vi "Leader.vi"   [LabVIEW 2016]
uses:
  <vilib>/NXT/Block Support/NXT_TimerIndex.ctl
  <vilib>/NXT/Block Support/NXT_OutputPort.ctl
  <vilib>/NXT/Subs/MotorOutput.ctl
  <vilib>/NXT/Dual Mode Library/Sensors/Reset_Timer.vi
  <vilib>/NXT/Dual Mode Library/Sensors/Read_Timer.vi
  <vilib>/NXT/Dual Mode Library/Motors/ResetMotor.vi
  <vilib>/NXT/Dual Mode Library/Motors/Rotation.vi
  <vilib>/NXT/NXTIO Xnodes/NXTIONodeSubVIs/NXTMoveMotors.vi
  <vilib>/NXT/Dual Mode Library/Display/drawNumber_float.vi
  <vilib>/NXT/NXTIO Xnodes/NXTIONodeSubVIs/NXTStopMotors.vi
  <vilib>/NXT/Dual Mode Library/Display/drawText.vi
  <vilib>/NXT/Dual Mode Library/Display/drawNumber.vi
  <vilib>/NXT/Dual Mode Library/Display/drawText_Right.vi
  <vilib>/NXT/Subs/LVHSConnector.ctl
  <vilib>/NXT/NXTIO Xnodes/AddressXNode/NXTIOAddress.xnode
  <vilib>/NXT/NXTIO Xnodes/NXTIOXNode/NXTIO.xnode
  <vilib>/NXT/LegoClasses/BrickReference/BrickReference.lvclass
types:
  T1 = typedef "NXT_TimerIndex.ctl" = u8
  T2 = typedef "LVHSConnector.ctl" = refnum<class "BrickReference.lvclass">
  T3 = typedef "NXT_OutputPort.ctl" = u8
  T4 = typedef "MotorOutput.ctl" = u8
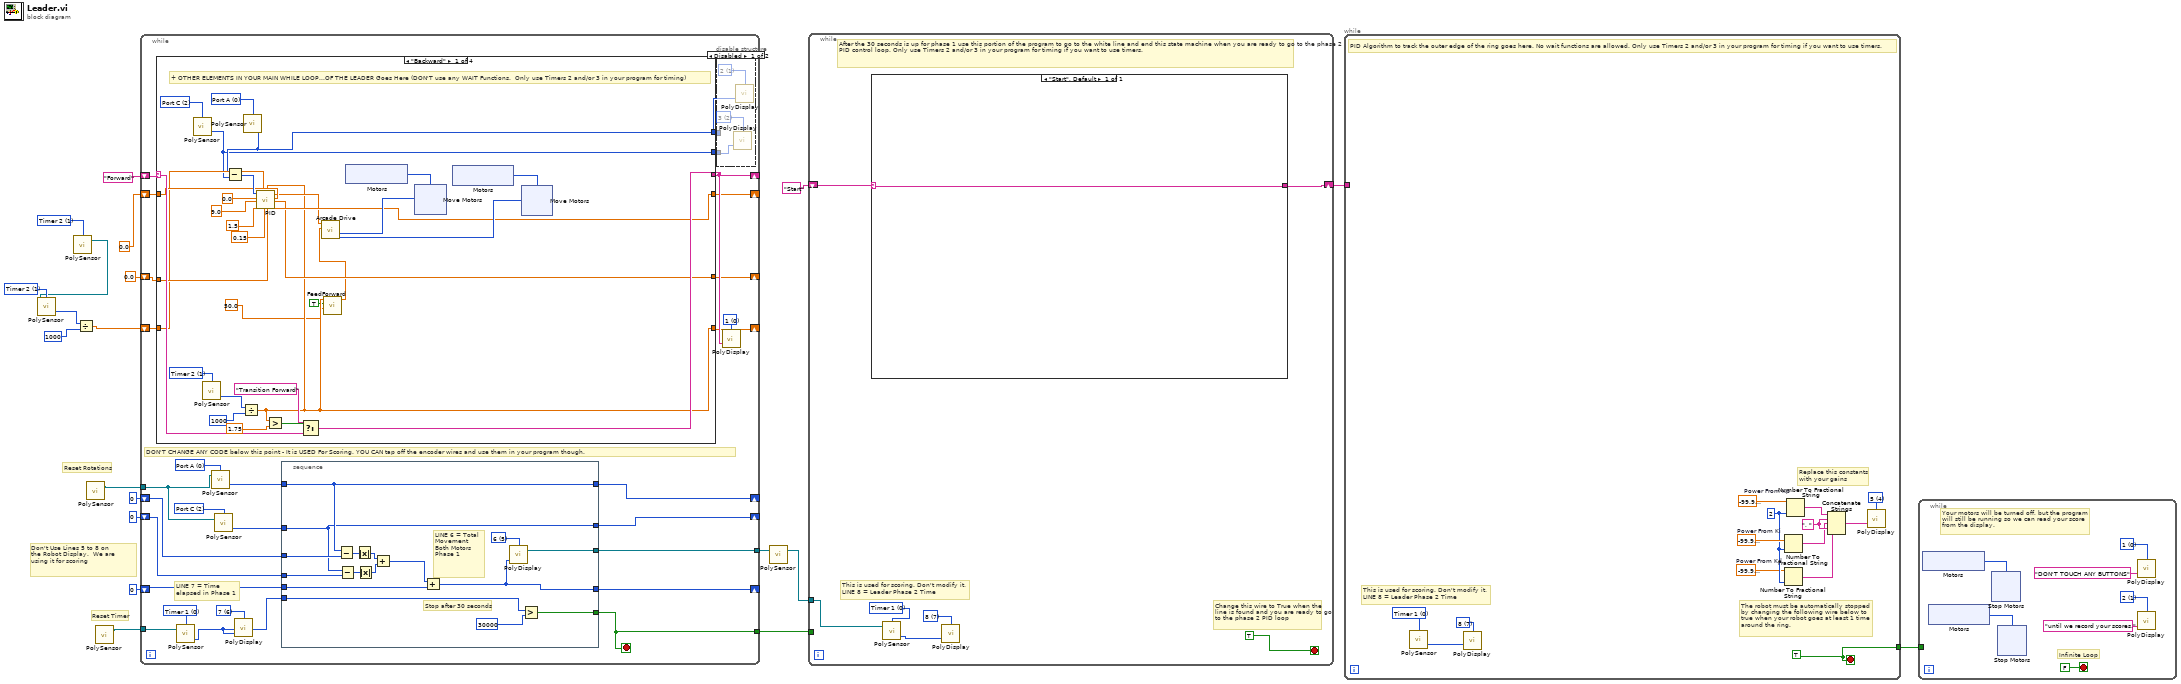
[diagram p0: block diagram]
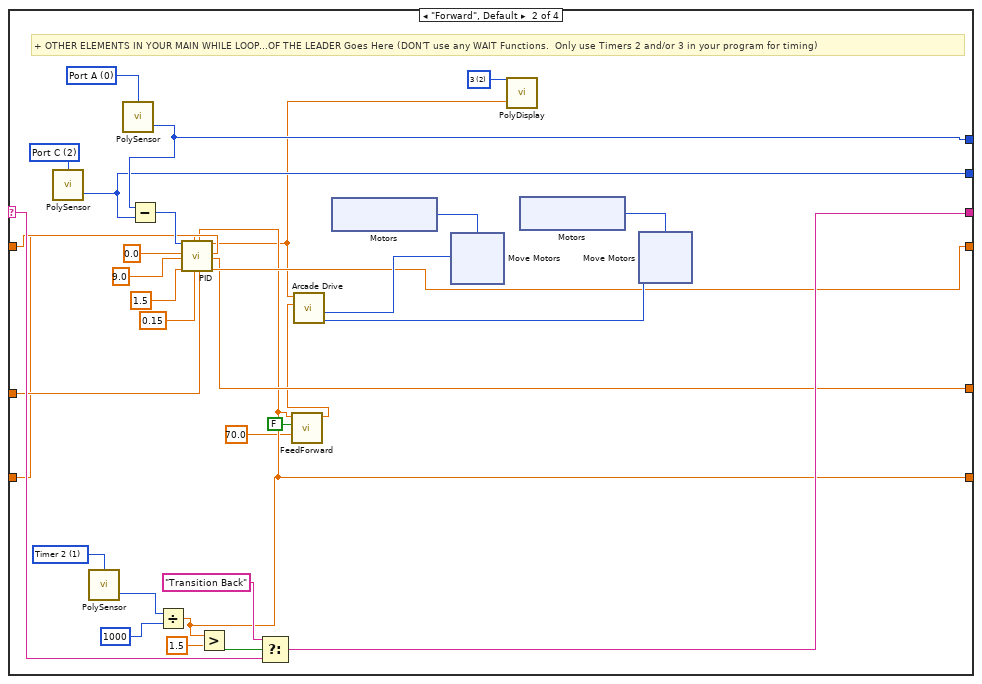
[diagram p3: hidden frame]
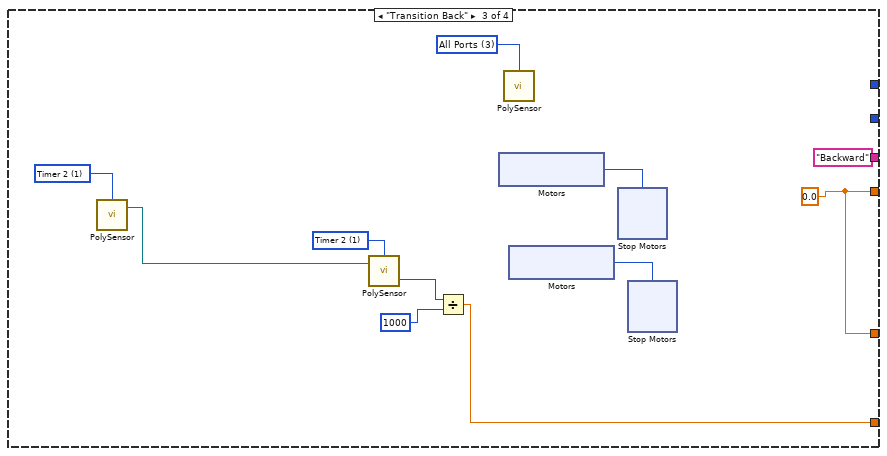
[diagram p4: hidden frame]
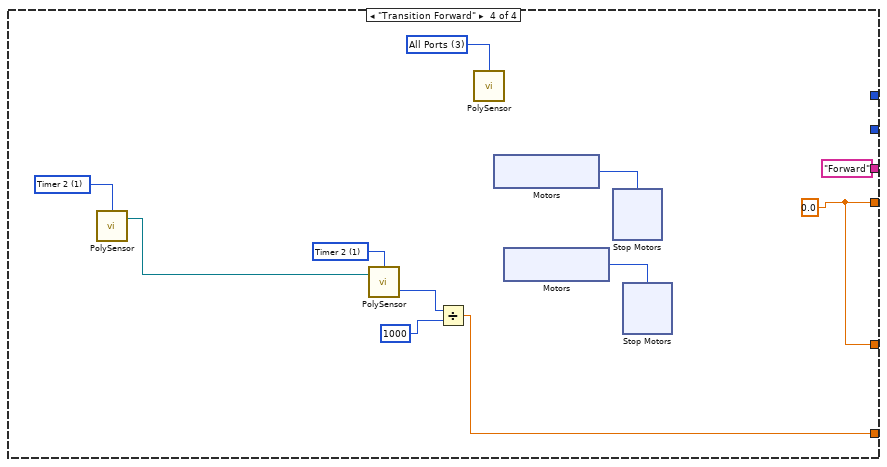
[diagram p5: hidden frame]
diagram:
  w4 = T1 1 items=["Timer 1", "Timer 2", "Timer 3"] ("Timer (Timer 1)")
  w8 = T1 1 items=["Timer 1", "Timer 2", "Timer 3"] ("Timer (Timer 1)")
  # "Don't Use Lines 5 to 8 on\nthe Robot Display.  We are \nusing it for scoring"
  # "Reset Timer"
  # "Reset Rotations"
  n1 = call-poly <vilib>:"PolySensor.vi"("Timer (Timer 1)"=w8) -> ("NXT/EV3"=w2:T2)  [unwired: 3 in]
  n2 = call-poly <vilib>:"PolySensor.vi"("NXT/EV3"=w2, "Timer (Timer 1)"=w4) -> ("Value (msec)"=w5:u32)  [unwired: 1 in, 1 out]
  n3 = Divide(x=w5, y=u32 1000) -> (x/y=w1:dbl)
  n4 = call-poly <vilib>:"PolySensor.vi"() -> ("NXT/EV3"=w16:T2)  [unwired: 4 in]
  n5 = call-poly <vilib>:"PolySensor.vi"() -> ("NXT/EV3"=w15:T2)  [unwired: 4 in]
  n6 = while {
    tunnel: w16 -> [w48]
    shift-right: [w40] -> _
    shift-left: 0 ("Angle of Rotation") -> [w42]
    shift-right: [w39] -> _
    shift-left: 0 ("Angle of Rotation") -> [w41]
    shift-right: [w46] -> _
    shift-left: 0 -> [w47]
    tunnel: w15 -> [w36]
    tunnel: [w45] -> w13
    shift-right: [w29] -> _
    shift-left: "Forward" -> [w38]
    tunnel: [w31] -> w12
    shift-right: [w27] -> _
    shift-left: 0.0 ("Accumulate In") -> [w28]
    shift-right: [w25] -> _
    shift-left: 0.0 ("Accumulate In") -> [w26]
    shift-right: [w23] -> _
    shift-left: w1 -> [w24]
    stop <- w45 stop-if-true
    w30 = i16 0 items=["1", "2", "3", "4", "5", "6", "7", "8", "9", "10", "11", "12"] ("Line")
    w33 = i16 6 items=["1", "2", "3", "4", "5", "6", "7", "8", "9", "10", "11", "12"] ("Line")
    w34 = T3 0 items=["Port A", "Port B", "Port C", "Port D"] ("Port (Port A)")
    w35 = T3 2 items=["Port A", "Port B", "Port C", "Port D"] ("Port (Port A)")
    w37 = T1 0 items=["Timer 1", "Timer 2", "Timer 3"] ("Timer (Timer 1)")
    # "DON'T CHANGE ANY CODE below this point - It is USED For Scoring. YOU CAN tap off the encoder wires and use them in your program though."
    # "LINE 7 = Time elapsed in Phase 1"
    n7 = case shown="\"Backward\"" w38 {
      selector: w38 -> [w78 w126 _ _]
      tunnel: [w79 w127 "Backward" ("t") "Forward" ("t")] -> w29
      tunnel: w28 -> [w65 w113 _ _]
      tunnel: [w63 w111 w156 w179] -> w27
      tunnel: w26 -> [w62 w110 _ _]
      tunnel: [w64 w112 w156 w179] -> w25
      tunnel: w24 -> [w61 w109 _ _]
      tunnel: [w57 w106 w151 w174] -> w23
      tunnel: [w60 w108 _ _] -> w22
      tunnel: [w59 w107 _ _] -> w21
      frame "Backward" {
        w73 = T3 2 items=["Port A", "Port B", "Port C", "Port D"] ("Port (Port A)")
        w74 = T3 0 items=["Port A", "Port B", "Port C", "Port D"] ("Port (Port A)")
        w81 = T1 1 items=["Timer 1", "Timer 2", "Timer 3"] ("Timer (Timer 1)")
        # "+ OTHER ELEMENTS IN YOUR MAIN WHILE LOOP...OF THE LEADER Goes Here (DON'T use any WAIT Functions.  Only use Timers 2 and/or 3 in your program for timing)"
        n8 = call-poly <vilib>:"PolySensor.vi"("Port (Port A)"=w73) -> ("Angle of Rotation"=w59:i32)  [unwired: 2 in, 1 out]
        n9 = call-poly <vilib>:"PolySensor.vi"("Timer (Timer 1)"=w81) -> ("Value (msec)"=w72:u32)  [unwired: 2 in, 1 out]
        n10 = Divide(x=w72, y=u32 1000) -> (x/y=w57:dbl)
        n11 = call-poly <vilib>:"PolySensor.vi"("Port (Port A)"=w74) -> ("Angle of Rotation"=w60:i32)  [unwired: 2 in, 1 out]
        n12 = Subtract(x=w60, y=w59) -> (x-y=w70:i32)
        n13 = call "PID.vi"("Sensor Input"=w70, "Setpoint"=0.0, "Kp"=9.0, "Ki"=1.5, "Prev Time"=w61, "Kd"=0.15, "Curr Time"=w57, "Accumulate In"=w65, "Previous Error"=w62) -> ("Output Val"=w58:dbl, "Accumulate Out"=w63:dbl, "Current Error"=w64:dbl)  [unwired: 5 in, 3 out]
        n14 = Greater?(x=w57, y=1.75) -> (0:w80:bool)
        n15 = Select(t="Transition Forward", s=w80, f=w78) -> (s? t:f=w79:string)
        n16 = call "FeedForward.vi"("FF Strength"=50.0, "backward?"=TRUE, "Current Time"=w57) -> ("f(t)"=w55:sgl)  [unwired: 8 in]
        n17 = call "Arcade Drive.vi"("Drive"=w55, "Rotate"=w58) -> ("Left Motor"=w75:i8, "Right Motor"=w76:i8)  [unwired: 8 in]
        n18 = xnode "Motors"() -> ("Motor"=w82:T3)
        n19 = xnode "Move Motors"("Power/Speed 1"=w76, "Motors"=w82) -> ()  [unwired: 1 in, 1 out]
        n20 = xnode "Motors"() -> ("Motor"=w83:T3)
        n21 = xnode "Move Motors"("Power/Speed 1"=w75, "Motors"=w83) -> ()  [unwired: 1 in, 1 out]
      }
      frame "Forward", Default {
        w103 = i16 2 items=["1", "2", "3", "4", "5", "6", "7", "8", "9", "10", "11", "12"] ("Line")
        w121 = T3 2 items=["Port A", "Port B", "Port C", "Port D"] ("Port (Port A)")
        w122 = T3 0 items=["Port A", "Port B", "Port C", "Port D"] ("Port (Port A)")
        w129 = T1 1 items=["Timer 1", "Timer 2", "Timer 3"] ("Timer (Timer 1)")
        # "+ OTHER ELEMENTS IN YOUR MAIN WHILE LOOP...OF THE LEADER Goes Here (DON'T use any WAIT Functions.  Only use Timers 2 and/or 3 in your program for timing)"
        n22 = call-poly <vilib>:"PolySensor.vi"("Port (Port A)"=w121) -> ("Angle of Rotation"=w107:i32)  [unwired: 2 in, 1 out]
        n23 = call-poly <vilib>:"PolySensor.vi"("Timer (Timer 1)"=w129) -> ("Value (msec)"=w120:u32)  [unwired: 2 in, 1 out]
        n24 = call-poly <vilib>:"PolySensor.vi"("Port (Port A)"=w122) -> ("Angle of Rotation"=w108:i32)  [unwired: 2 in, 1 out]
        n25 = Subtract(x=w108, y=w107) -> (x-y=w118:i32)
        n26 = Divide(x=w120, y=u32 1000) -> (x/y=w106:dbl)
        n27 = call "PID.vi"("Sensor Input"=w118, "Setpoint"=0.0, "Kp"=9.0, "Ki"=1.5, "Prev Time"=w109, "Kd"=0.15, "Curr Time"=w106, "Accumulate In"=w113, "Previous Error"=w110) -> ("Output Val"=w104:dbl, "Accumulate Out"=w111:dbl, "Current Error"=w112:dbl)  [unwired: 5 in, 3 out]
        n28 = Greater?(x=w106, y=1.5) -> (0:w128:bool)
        n29 = Select(t="Transition Back", s=w128, f=w126) -> (s? t:f=w127:string)
        n30 = call "FeedForward.vi"("FF Strength"=70.0, "backward?"=FALSE, "Current Time"=w106) -> ("f(t)"=w102:sgl)  [unwired: 8 in]
        n31 = call "Arcade Drive.vi"("Drive"=w102, "Rotate"=w104) -> ("Left Motor"=w123:i8, "Right Motor"=w124:i8)  [unwired: 8 in]
        n32 = xnode "Motors"() -> ("Motor"=w130:T3)
        n33 = xnode "Move Motors"("Power/Speed 1"=w124, "Motors"=w130) -> ()  [unwired: 1 in, 1 out]
        n34 = call-poly <vilib>:"PolyDisplay.vi"("number"=w104, "Line"=w103) -> ()  [unwired: 2 in, 1 out]
        n35 = xnode "Motors"() -> ("Motor"=w131:T3)
        n36 = xnode "Move Motors"("Power/Speed 1"=w123, "Motors"=w131) -> ()  [unwired: 1 in, 1 out]
      }
      frame "Transition Back" {
        w150 = T4 3 items=["Port A"=0, "Port B"=1, "Port C"=2, "Ports A & B"=4, "Ports A & C"=5, "Ports B & C"=6, "All Ports"=3] ("Port (All Ports)")
        w154 = T1 1 items=["Timer 1", "Timer 2", "Timer 3"] ("Timer (Timer 1)")
        w156 = 0.0 ("Accumulate In")
        w158 = T1 1 items=["Timer 1", "Timer 2", "Timer 3"] ("Timer (Timer 1)")
        n37 = call-poly <vilib>:"PolySensor.vi"("Timer (Timer 1)"=w158) -> ("NXT/EV3"=w152:T2)  [unwired: 3 in]
        n38 = call-poly <vilib>:"PolySensor.vi"("NXT/EV3"=w152, "Timer (Timer 1)"=w154) -> ("Value (msec)"=w153:u32)  [unwired: 1 in, 1 out]
        n39 = Divide(x=w153, y=u32 1000) -> (x/y=w151:dbl)
        n40 = xnode "Motors"() -> ("Motor"=w149:T3)
        n41 = call-poly <vilib>:"PolySensor.vi"("Port (All Ports)"=w150) -> ()  [unwired: 3 in, 1 out]
        n42 = xnode "Motors"() -> ("Motor"=w148:T3)
        n43 = xnode "Stop Motors"("Motors"=w149) -> ()  [unwired: 1 in, 1 out]
        n44 = xnode "Stop Motors"("Motors"=w148) -> ()  [unwired: 1 in, 1 out]
      }
      frame "Transition Forward" {
        w173 = T4 3 items=["Port A"=0, "Port B"=1, "Port C"=2, "Ports A & B"=4, "Ports A & C"=5, "Ports B & C"=6, "All Ports"=3] ("Port (All Ports)")
        w177 = T1 1 items=["Timer 1", "Timer 2", "Timer 3"] ("Timer (Timer 1)")
        w179 = 0.0 ("Accumulate In")
        w181 = T1 1 items=["Timer 1", "Timer 2", "Timer 3"] ("Timer (Timer 1)")
        n45 = call-poly <vilib>:"PolySensor.vi"("Timer (Timer 1)"=w181) -> ("NXT/EV3"=w175:T2)  [unwired: 3 in]
        n46 = call-poly <vilib>:"PolySensor.vi"("NXT/EV3"=w175, "Timer (Timer 1)"=w177) -> ("Value (msec)"=w176:u32)  [unwired: 1 in, 1 out]
        n47 = Divide(x=w176, y=u32 1000) -> (x/y=w174:dbl)
        n48 = call-poly <vilib>:"PolySensor.vi"("Port (All Ports)"=w173) -> ()  [unwired: 3 in, 1 out]
        n49 = xnode "Motors"() -> ("Motor"=w172:T3)
        n50 = xnode "Motors"() -> ("Motor"=w171:T3)
        n51 = xnode "Stop Motors"("Motors"=w172) -> ()  [unwired: 1 in, 1 out]
        n52 = xnode "Stop Motors"("Motors"=w171) -> ()  [unwired: 1 in, 1 out]
      }
    }
    n53 = call-poly <vilib>:"PolySensor.vi"("NXT/EV3"=w36, "Timer (Timer 1)"=w37) -> ("Value (msec)"=w32:u32)  [unwired: 1 in, 1 out]
    n54 = call-poly <vilib>:"PolySensor.vi"("NXT/EV3"=w48, "Port (Port A)"=w34) -> ("Angle of Rotation"=w44:i32)  [unwired: 1 in, 1 out]
    n55 = call-poly <vilib>:"PolySensor.vi"("NXT/EV3"=w48, "Port (Port A)"=w35) -> ("Angle of Rotation"=w43:i32)  [unwired: 1 in, 1 out]
    n56 = call-poly <vilib>:"PolyDisplay.vi"("number"=w32, "Line"=w33) -> ()  [unwired: 2 in, 1 out]
    n57 = stacked-sequence {
      tunnel: w47 -> [w209]
      tunnel: [w196] -> w46
      tunnel: w32 -> [w207]
      tunnel: [w206] -> w45
      tunnel: w44 -> [w199]
      tunnel: w43 -> [w198]
      tunnel: w42 -> [w201]
      tunnel: w41 -> [w200]
      tunnel: [w199] -> w40
      tunnel: [w198] -> w39
      tunnel: [w194] -> w31
      frame #0 {
        w195 = i16 5 items=["1", "2", "3", "4", "5", "6", "7", "8", "9", "10", "11", "12"] ("Line")
        # "LINE 6 = Total\nMovement\nBoth Motors\nPhase 1"
        # "Stop after 30 seconds"
        n58 = Subtract(x=w199, y=w201) -> (x-y=w205:i32)
        n59 = Subtract(x=w198, y=w200) -> (x-y=w204:i32)
        n60 = Absolute Value(x=w205) -> (abs(x)=w203:i32)
        n61 = Absolute Value(x=w204) -> (abs(x)=w202:i32)
        n62 = Add(x=w203, y=w202) -> (x+y=w197:i32)
        n63 = Add(x=w197, y=w209) -> (x+y=w196:i32)
        n64 = call-poly <vilib>:"PolyDisplay.vi"("number"=w196, "Line"=w195) -> ("NXT/EV3"=w194:T2)  [unwired: 2 in]
        n65 = Greater?(x=w207, y=u32 30000 ("Value (msec)")) -> (0:w206:bool)
      }
    }
    n66 = disable-structure shown="Disabled" {
      disable-tunnel: w22 -> [w51 _]
      disable-tunnel: w21 -> [w49 _]
      frame Disabled {
        w50 = i16 2 items=["1", "2", "3", "4", "5", "6", "7", "8", "9", "10", "11", "12"] ("Line")
        w52 = i16 1 items=["1", "2", "3", "4", "5", "6", "7", "8", "9", "10", "11", "12"] ("Line")
        n67 = call-poly <vilib>:"PolyDisplay.vi"("number"=w49, "Line"=w50) -> ()  [unwired: 2 in, 1 out]
        n68 = call-poly <vilib>:"PolyDisplay.vi"("number"=w51, "Line"=w52) -> ()  [unwired: 2 in, 1 out]
      }
      frame Enabled {
      }
    }
    n69 = call-poly <vilib>:"PolyDisplay.vi"("Text"=w29, "Line"=w30) -> ()  [unwired: 2 in, 1 out]
  }
  n70 = call-poly <vilib>:"PolySensor.vi"("NXT/EV3"=w12) -> ("NXT/EV3"=w11:T2)  [unwired: 3 in]
  n71 = while {
    shift-right: [w215] -> w10
    shift-left: "Start" -> [w216]
    tunnel: w13 -> [_]
    tunnel: w11 -> [w211]
    stop <- TRUE stop-if-true
    w213 = i16 7 items=["1", "2", "3", "4", "5", "6", "7", "8", "9", "10", "11", "12"] ("Line")
    w214 = T1 0 items=["Timer 1", "Timer 2", "Timer 3"] ("Timer (Timer 1)")
    # "This is used for scoring. Don't modify it.\nLINE 8 = Leader Phase 2 Time"
    # "Change this wire to True when the line is found and you are ready to go to the phase 2 PID loop"
    # "After the 30 seconds is up for phase 1 use this portion of the program to go to the white line and end this state machine when you are ready to go to the phase 2 PID control loop. Only use Timers 2 and/or 3 in your program for timing if you want to use timers."
    n72 = case shown="\"Start\", Default" w216 {
      selector: w216 -> [w217]
      tunnel: [w217] -> w215
      frame "Start", Default {
      }
    }
    n73 = call-poly <vilib>:"PolySensor.vi"("NXT/EV3"=w211, "Timer (Timer 1)"=w214) -> ("Value (msec)"=w212:u32)  [unwired: 1 in, 1 out]
    n74 = call-poly <vilib>:"PolyDisplay.vi"("number"=w212, "Line"=w213) -> ()  [unwired: 2 in, 1 out]
  }
  n75 = while {
    tunnel: [w228] -> w9
    tunnel: w10 -> [_]
    stop <- w228 stop-if-true
    w221 = ", " ("string")
    w224 = i16 2 ("precision (6)")
    w223 = sgl -99.9  # Power From Kd
    w225 = sgl -99.9  # Power From Ki
    w226 = sgl -99.9  # Power From Kp
    w227 = i16 4 items=["1", "2", "3", "4", "5", "6", "7", "8", "9", "10", "11", "12"] ("Line")
    w228 = TRUE
    w229 = i16 7 items=["1", "2", "3", "4", "5", "6", "7", "8", "9", "10", "11", "12"] ("Line")
    w231 = T1 0 items=["Timer 1", "Timer 2", "Timer 3"] ("Timer (Timer 1)")
    # "Replace this constants\nwith your gains"
    # "This is used for scoring. Don't modify it.\nLINE 8 = Leader Phase 2 Time"
    # "The robot must be automatically stopped\nby changing the following wire below to\ntrue when your robot goes at least 1 time\naround the ring."
    # "PID Algorithm to track the outer edge of the ring goes here. No wait functions are allowed. Only use Timers 2 and/or 3 in your program for timing if you want to use timers."
    n76 = call-poly <vilib>:"PolySensor.vi"("Timer (Timer 1)"=w231) -> ("Value (msec)"=w230:u32)  [unwired: 2 in, 1 out]
    n77 = call-poly <vilib>:"PolyDisplay.vi"("number"=w230, "Line"=w229) -> ()  [unwired: 2 in, 1 out]
    n78 = Number To Fractional String(number=w225, precision (6)=w224) -> (F-format string=w220:string)  [unwired: 2 in]
    n79 = Number To Fractional String(number=w223, precision (6)=w224) -> (F-format string=w219:string)  [unwired: 2 in]
    n80 = Number To Fractional String(number=w226, precision (6)=w224) -> (F-format string=w222:string)  [unwired: 2 in]
    n81 = Concatenate Strings(w222, w221, w220, w221, w219) -> (w218:string)
    n82 = call-poly <vilib>:"PolyDisplay.vi"("Text"=w218, "Line"=w227) -> ()  [unwired: 2 in, 1 out]
  }
  n83 = while {
    tunnel: w9 -> [_]
    stop <- FALSE stop-if-true
    w235 = i16 1 items=["1", "2", "3", "4", "5", "6", "7", "8", "9", "10", "11", "12"] ("Line")
    w234 = i16 0 items=["1", "2", "3", "4", "5", "6", "7", "8", "9", "10", "11", "12"] ("Line")
    # "Your motors will be turned off, but the program\nwill still be running so we can read your score\nfrom the display."
    # "Infinite Loop"
    n84 = xnode "Motors"() -> ("Motor"=w237:T3)
    n85 = xnode "Motors"() -> ("Motor"=w236:T3)
    n86 = xnode "Stop Motors"("Motors"=w237) -> ()  [unwired: 1 in, 1 out]
    n87 = xnode "Stop Motors"("Motors"=w236) -> ()  [unwired: 1 in, 1 out]
    n88 = call-poly <vilib>:"PolyDisplay.vi"("Text"="DON'T TOUCH ANY BUTTONS", "Line"=w234) -> ()  [unwired: 2 in, 1 out]
    n89 = call-poly <vilib>:"PolyDisplay.vi"("Text"="until we record your scores.", "Line"=w235) -> ()  [unwired: 2 in, 1 out]
  }
